vi "initialise.vi"(8 "error in (no error)":errorcluster, 11 "MG090622IMAQCamera in":refnum<class "DAQ_MG090622Camera.lvclass">) -> (0 "error out":errorcluster, 3 "MG090622IMAQCamera out":refnum<class "DAQ_MG090622Camera.lvclass">)   [LabVIEW 2010, in "DAQ_MG090622Camera.lvclass"]
doc: "The dynamic dispatch-version of this VI initalises the plug-in object by allocating and initalising any dynamic resources need."
uses:
  DAQ_MG090622Camera.lvclass
  DAQ_DL090211Scaffold/DAQ_DL090211Scaffold/DAQ_DL090211Scaffold.lvclass
  DAQ_MG090622Camera.lvclass/DAQ_MG090622Camera.ctl
  <vilib>/userDefined/High Color/IMAQdx.ctl
  common/classes/Image/Image/Image.lvclass
  common/classes/ErrorController/ErrorController/class_data.vi
  common/classes/ErrorController/ErrorController/ErrorController.lvclass
  <vilib>/vision/driver/NI_Vision_Acquisition_Software.lvlib
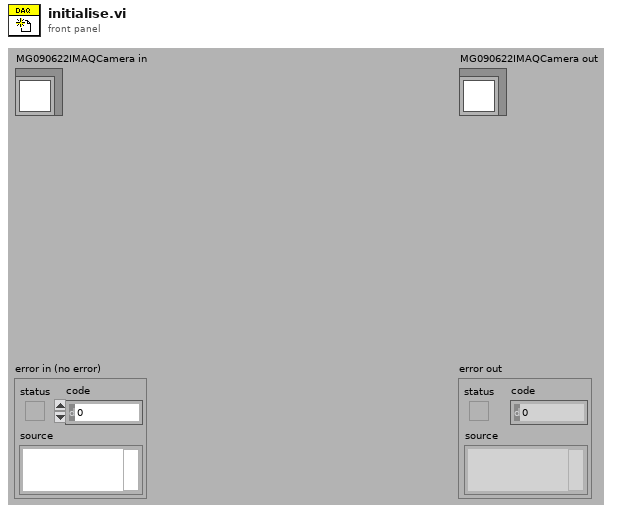
[diagram p1: front panel]
types:
  T1 = typedef "IMAQdx.ctl" = refnum<k21>
  T2 = typedef "DAQ_MG090622Camera.lvclass/camera_type_enum.ctl" = enum16{"gray scale", "RGB"}
  T3 = typedef "DAQ_MG090622Camera.lvclass/connection_type_enum.ctl" = enum16{"IEEE 1394 (FireWire)", "USB", "GigE", "CameraLink"}
  T4 = typedef "Image Type" = u32
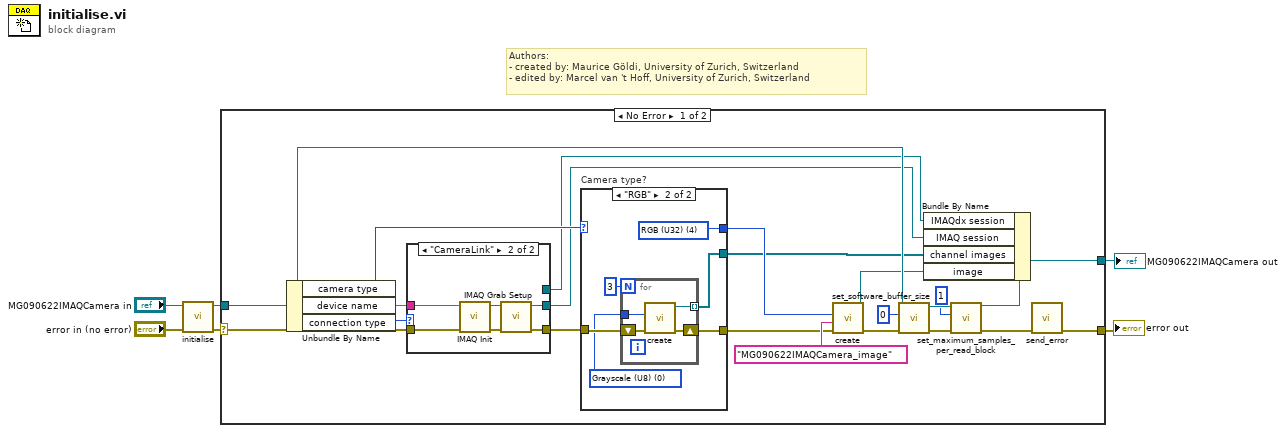
[diagram p0: block diagram]
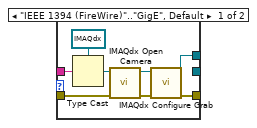
[diagram p2: hidden frame]
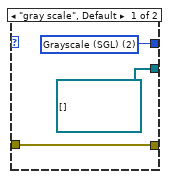
[diagram p3: hidden frame]
diagram:
  # "Authors: \n- created by: Maurice Göldi, University of Zurich, Switzerland\n- edited by: Marcel van 't Hoff, University of Zurich, Switzerland"
  n1 = call-parent "initialise.vi"("error in (no error)"="error in (no error)", "GenericPlugin in"="MG090622IMAQCamera in") -> ("error out"=w4:errorcluster, "GenericPlugin out"=w1:refnum<class "DAQ_MG090622Camera.lvclass">)  [unwired: 8 out]
  n2 = case shown="No Error" w4 {
    selector: w4 -> [w26 w57]
    tunnel: [w9 w57] -> w6
    tunnel: w1 -> [w22 w56]
    tunnel: [w27 w56] -> w5
    frame No Error {
      n3 = Unbundle By Name(w22) -> ("camera type"=w18:T2, "device name"=w28:string, "connection type"=w8:T3)
      n4 = case shown="\"CameraLink\"" w8 {
        tunnel: w28 -> [w32 w38]
        tunnel: w26 -> [w34 w41]
        tunnel: [w33 w39] -> w25
        tunnel: [_ w37] -> w12
        tunnel: [w29 _] -> w7
        frame "IEEE 1394 (FireWire)".."GigE", Default {
          n5 = Type Cast(type=T1 refnum ("Session In"), x=w32) -> (*(type *) &x=w30:T1)
          n6 = call <vilib>:"IMAQdx Open Camera.vi"("error in"=w34, "Session In"=w30) -> ("error out"=w36:errorcluster, "Session Out"=w35:T1)  [unwired: 8 in]
          n7 = call <vilib>:"IMAQdx Configure Grab.vi"("error in"=w36, "Session In"=w35) -> ("error out"=w33:errorcluster, "Session Out"=w29:T1)  [unwired: 8 in]
        }
        frame "CameraLink" {
          n8 = call <vilib>:"IMAQ Init.vi"("error in (no error)"=w41, "Interface Name"=w38) -> ("error out"=w40:errorcluster, "IMAQ Session Out"=w42:refnum<k11>)  [unwired: 8 out]
          n9 = call <vilib>:"IMAQ Grab Setup.vi"("error in (no error)"=w40, "IMAQ Session In"=w42) -> ("error out"=w39:errorcluster, "IMAQ Session Out"=w37:refnum<k11>)  [unwired: 8 out]
        }
      }
      n10 = case "Camera type?" shown="\"RGB\"" w18 {
        tunnel: w25 -> [w45 w48]
        tunnel: [w45 w47] -> w15
        tunnel: [w43 w51] -> w16
        tunnel: [refnum<class "Image.lvclass">[] [] w50] -> w13
        frame "gray scale", Default {
          w43 = T4 2 items=["Grayscale (U8)", "Grayscale (I16)", "Grayscale (SGL)", "Complex (CSG)", "RGB (U32)", "HSL (U32)", "RGB (U64)", "Grayscale (U16)"] ("Image Type")
        }
        frame "RGB" {
          w46 = T4 0 items=["Grayscale (U8)", "Grayscale (I16)", "Grayscale (SGL)", "Complex (CSG)", "RGB (U32)", "HSL (U32)", "RGB (U64)", "Grayscale (U16)"] ("Image Type")
          w51 = T4 4 items=["Grayscale (U8)", "Grayscale (I16)", "Grayscale (SGL)", "Complex (CSG)", "RGB (U32)", "HSL (U32)", "RGB (U64)", "Grayscale (U16)"] ("Image Type")
          n11 = for {
            N: 3 -> [_]
            tunnel: w46 -> [w55]
            tunnel: [w54] -> w50 mode=indexing
            shift-right: [w52] -> w47
            shift-left: w48 -> [w53]
            n12 = call "create.vi"("error in (no error)"=w53, "Image Type"=w55) -> ("error out"=w52:errorcluster, "Image out"=w54:refnum<class "Image.lvclass">)  [unwired: 2 in, 6 out]
          }
        }
      }
      n13 = call "create.vi"("error in (no error)"=w15, "name"="MG090622IMAQCamera_image", "Image Type"=w16) -> ("error out"=w14:errorcluster, "Image out"=w11:refnum<class "Image.lvclass">)  [unwired: 1 in, 6 out]
      n14 = call-dynamic "set_software_buffer_size.vi"("error in (no error)"=w14, "software buffer size"=0, "GenericDAQ.lvclass in"=w22) -> ("error out"=w24:errorcluster, "GenericDAQ.lvclass out"=w23:refnum<class "DAQ_MG090622Camera.lvclass">)  [unwired: 7 out]
      n15 = call-dynamic "set_maximum_samples_per_read_block.vi"("error in (no error)"=w24, "samples per block"=1, "GenericDAQ.lvclass in"=w23) -> ("error out"=w10:errorcluster, "GenericDAQ.lvclass out"=w21:refnum<class "DAQ_MG090622Camera.lvclass">)  [unwired: 7 out]
      n16 = Bundle By Name(cluster=w21, "IMAQdx session"=w7, "IMAQ session"=w12, "channel images"=w13, "image"=w11) -> (w27:refnum<class "DAQ_MG090622Camera.lvclass">)
      n17 = call "send_error.vi"("error in (no error)"=w10) -> ("error out"=w9:errorcluster)  [unwired: 10 in]
    }
    frame Error {
    }
  }
  "error out" <- w6
  "MG090622IMAQCamera out" <- w5
